vi "Close VI Server Application Control Event.vi"(8 "error in (no error)":errorcluster, 11 "VI refnum":refnum<vi>) -> (0 "error out":errorcluster)   [LabVIEW 2012]
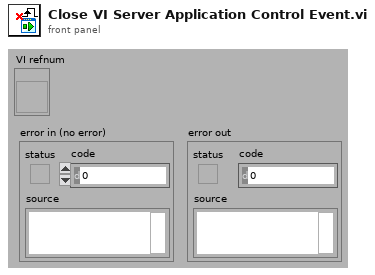
[diagram p1: front panel]
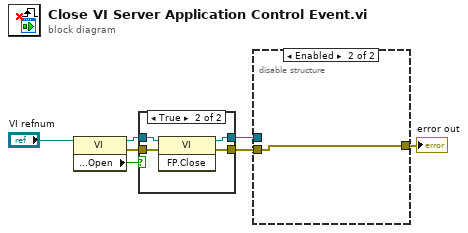
[diagram p0: block diagram]
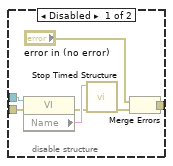
[diagram p2: hidden frame]
diagram:
  n1 = property class="VI"(reference="VI refnum") -> (reference out=w2:refnum<vi>, error out=w3:errorcluster, "Front Panel.Open"=w1:bool)  [unwired: 1 in]
  n2 = case shown="True" w1 {
    tunnel: [w9 w13] -> w5
    tunnel: [w8 w12] -> w6
    tunnel: w2 -> [w9 w11]
    tunnel: w3 -> [w8 w10]
    frame False {
    }
    frame True {
      n3 = invoke class="VI" method="FP.Close"(reference=w11, error in=w10) -> (reference out=w13:refnum<vi>, error out=w12:errorcluster)  [unwired: 1 in, 1 out]
    }
  }
  n4 = disable-structure shown="Enabled" {
    disable-tunnel: w6 -> [w20 w21]
    disable-tunnel: w5 -> [w19 _]
    disable-tunnel: [w18 w21] -> w4
    frame Disabled {
      n5 = property class="VI"(reference=w19, error in=w20) -> (error out=w15:errorcluster, "Name"=w16:string)  [unwired: 1 out]
      n6 = call <vilib>:"Stop Timed Structure.vi"("error in (no error)"=w15, "name"=w16) -> ("error out"=w14:errorcluster)  [unwired: 9 in]
      n7 = Merge Errors("error in (no error)", w14) -> (w18:errorcluster)
    }
    frame Enabled {
    }
  }
  "error out" <- w4
